vi "16_Helper_CleanUp.vi"(8 "Error In":errorcluster) -> (0 "Error Out":errorcluster)   [LabVIEW 2020, in "16_Helper.lvclass"]
uses:
  16_Helper.lvclass
  16_Helper.lvclass/16_Helper.ctl
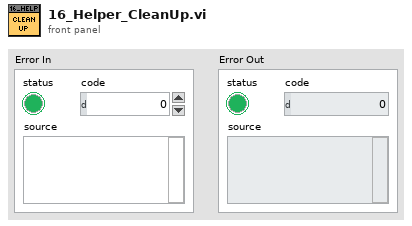
[diagram p1: front panel]
types:
  T1 = typedef "16_Helper.lvclass/ObjectAttributes.ctl" = cluster{"VersionNumberSum":u64}
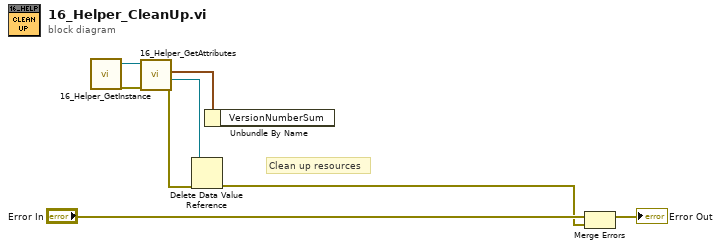
[diagram p0: block diagram]
diagram:
  # "Clean up resources"
  n1 = call "16_Helper_GetInstance.vi"() -> ("error out"=w6:errorcluster, "reference out"=w5:refnum<class "16_Helper.lvclass">)  [unwired: 7 in, 3 out]
  n2 = call "16_Helper_GetAttributes.vi"("error in (no error)"=w6, "reference in"=w5) -> ("error out"=w4:errorcluster, "DataRef"=w3:refnum<data-value>, "Data"=w7:T1)  [unwired: 6 in, 1 out]
  n3 = Delete Data Value Reference(data value reference=w3, error in=w4) -> (error out=w1:errorcluster)  [unwired: 1 out]
  n4 = Unbundle By Name(w7) -> ()  [unwired: 1 out]
  n5 = Merge Errors("Error In", w1) -> (→"Error Out":errorcluster)
